vi "Get Magnet Vector.vi"(8 "error in (no error)":errorcluster, 11 "Instrument.VRM in":refnum<class "Instrument.OxfordVRM.lvclass">) -> (0 "error out":errorcluster, 1 "status":string, 2 "Magnet Field (T)":dbl[](array[numeric]), 3 "Instrument.VRM out":refnum<class "Instrument.OxfordVRM.lvclass">, 4 "finished":bool)   [LabVIEW 2019, in "Instrument.OxfordVRM.lvclass"]
uses:
  Instrument.OxfordVRM.lvclass
  C:/Program Files (x86)/National Instruments/LabVIEW 2019/user.lib/LevyLab/Instrument Framework/Instrument/Instrument.lvclass
  Get Vector Magnet.vi/5e873d59-b7fa-4b76-b36a-7150f831c1b5.vi/1bc81592-5c83-492a-87df-01270eabf915.vi
  Get Vector Magnet.vi/5e873d59-b7fa-4b76-b36a-7150f831c1b5.vi/1bc81592-5c83-492a-87df-01270eabf915.vi/49bdcdb8-5a27-4d24-8450-55524beb0a43.vi
  Get Vector Magnet.vi/5e873d59-b7fa-4b76-b36a-7150f831c1b5.vi/1bc81592-5c83-492a-87df-01270eabf915.vi/a016e083-46fc-4635-8afd-7d2064752788.vi
  <userlib>/LevyLab/Instrument Framework/Instrument/API/Remote Client.vi
  <vilib>/Utility/Data Type/Get Type Information.vi
  <vilib>/JDP Science/JSONtext/JSON text to Variant.vi
  <vilib>/JDP Science/JSONtext/LVClass Serializer/JSONtext LVClass Serializer.lvclass
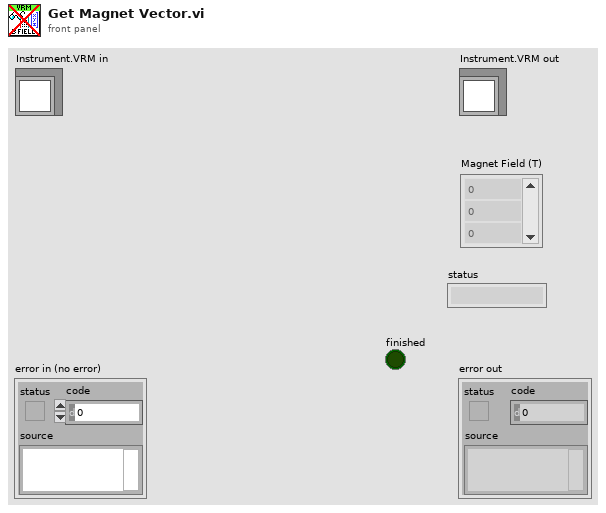
[diagram p1: front panel]
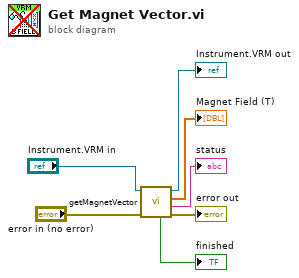
[diagram p0: block diagram]
diagram:
  n1 = call-dynamic "getMagnetVector.vi"("error in (no error)"="error in (no error)", "Instrument.VRM in"="Instrument.VRM in") -> ("error out"=→"error out":errorcluster, "status"=→"status":string, "Magnet Field (T)"=→"Magnet Field (T)":dbl[], "Instrument.VRM out"=→"Instrument.VRM out":refnum<class "Instrument.OxfordVRM.lvclass">, "finished"=→"finished":bool)  [unwired: 5 in]
